vi "Ismatec ISM831C Test Program.vi"() -> ()   [LabVIEW 2018, in "Ismatec ISM 831C.lvlib"]
uses:
  Ismatec ISM 831C.lvlib
  Controls/Ismatech Settings Cluster.ctl
panel:
  in  "stop":bool
  out "Connection Error 2":bool
  out "Pump On?":enum16{"Off", "On", "Not Initialized"}(ring)
  out "Connection Error":bool
  in  "Speed (%)":dbl
  out "error out":errorcluster
  in  "error in (no error)":errorcluster
  out "Ismatech Settings":T1={"VISA resource name"="", "Simulated?"=TRUE, "Pump Number"=1.0, "Reverse?"=FALSE} {"Pump Number" min=1.0 max=20.0 step=1.0}
  in  "Ismatech Settings":T1={"VISA resource name"="", "Simulated?"=TRUE, "Pump Number"=1.0, "Reverse?"=FALSE} {"Pump Number" min=1.0 max=20.0 step=1.0}
  in  "Pause":bool
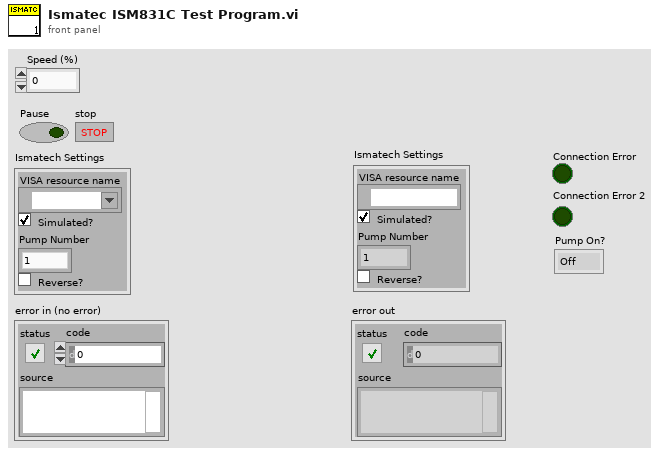
[diagram p1: front panel]
types:
  T1 = typedef "Ismatec ISM 831C.lvlib/Ismatech Settings Cluster.ctl" = cluster{"VISA resource name":refnum<visa-resource-name>, "Simulated?":bool, "Pump Number":dbl, "Reverse?":bool}
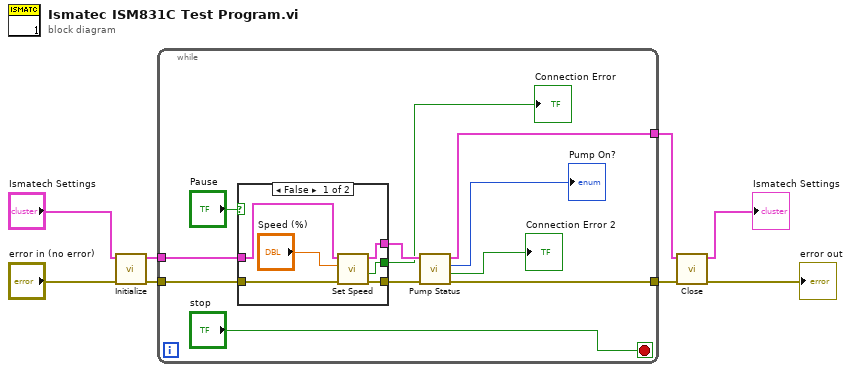
[diagram p0: block diagram]
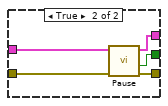
[diagram p2: hidden frame]
diagram:
  n1 = call "Initialize.vi"("error in (no error)"="error in (no error)", "Ismatech Settings"="Ismatech Settings") -> ("error out"=w5:errorcluster, "Ismatech Settings"=w6:T1)  [unwired: 6 in, 2 out]
  n2 = while {
    tunnel: w6 -> [w18]
    tunnel: w5 -> [w17]
    tunnel: [w14] -> w4
    tunnel: [w13] -> w2
    stop <- "stop" stop-if-true
    n3 = case shown="False" "Pause" {
      tunnel: w18 -> [w25 w30]
      tunnel: w17 -> [w24 w29]
      tunnel: [w22 w28] -> w16
      tunnel: [w21 w27] -> w15
      tunnel: [w20 w26] -> w12
      frame False {
        n4 = call "Set Speed.vi"("error in (no error)"=w24, "Speed (%)"="Speed (%)", "Ismatech Settings In"=w25) -> ("error out"=w21:errorcluster, "Connection Error"=w20:bool, "Ismatech Settings Out"=w22:T1)  [unwired: 6 in]
      }
      frame True {
        n5 = call "Pause.vi"("error in (no error)"=w29, "Ismatech Settings In"=w30) -> ("error out"=w27:errorcluster, "Connection Error"=w26:bool, "Ismatech Settings Out"=w28:T1)  [unwired: 7 in]
      }
    }
    "Connection Error" <- w12
    n6 = call "Pump Status.vi"("error in (no error)"=w15, "Ismatech Settings In"=w16) -> ("error out"=w13:errorcluster, "Connection Error"=→"Connection Error 2":bool, "Pump On?"=→"Pump On?":enum16{"Off", "On", "Not Initialized"}, "Ismatech Settings Out"=w14:T1)  [unwired: 6 in]
  }
  n7 = call "Close.vi"("error in (no error)"=w2, "Ismatech Settings"=w4) -> ("error out"=→"error out":errorcluster, "Ismatech Settings"=→"Ismatech Settings":T1)  [unwired: 7 in, 1 out]
